vi "get integrated iq from h5.vi"(8 "error in (no error)":errorcluster, 11 "path":path=path "C:/Users/dvh-collab-user/Desktop/20230313 Robert sample/tmp.hdf5") -> (0 "error out":errorcluster, 3 "Data out":dbl[][](array[numeric]))   [LabVIEW 2023]
uses:
  <vilib>/UPVI/lvhdf5/library.llb/HDF5 Ref.ctl
  <vilib>/UPVI/lvhdf5/dataset.llb/Read Dataset and All Attributes.xnode
  <vilib>/Utility/miscctls.llb/LVRectTypeDef.ctl
  <vilib>/UPVI/lvhdf5/file.llb/H5Fopen.vi
  <vilib>/UPVI/lvhdf5/group.llb/H5G_obj_t.ctl
  <vilib>/UPVI/lvhdf5/dataset.llb/LVH5D Operation.ctl
  <vilib>/UPVI/lvhdf5/file.llb/LVH5F Operation.ctl
  <vilib>/UPVI/lvhdf5/utility.llb/Select HDF5 Dialog.vi
  <vilib>/UPVI/lvhdf5/utility.llb/Select HDF5 Dialog (File and Object).vi
  <vilib>/UPVI/lvhdf5/utility.llb/Select HDF5 Dialog (Object Only).vi
  <vilib>/UPVI/lvhdf5/identifier.llb/Not an HDF5 Refnum Constant.vi
  <vilib>/UPVI/lvhdf5/dataset.llb/Simple H5Dread (Variant).vi
  <vilib>/UPVI/lvhdf5/dataset.llb/OpenCreateReplace Dataset.vi
  <vilib>/UPVI/lvhdf5/dataset.llb/H5Dget_space.vi
  <vilib>/UPVI/lvhdf5/dataspace.llb/H5Sget_simple_extent_dims.vi
  <vilib>/UPVI/lvhdf5/dataspace.llb/H5Sselect_hyperslab.vi
  <vilib>/UPVI/lvhdf5/dataset.llb/H5Dread (Variant).vi
  <vilib>/UPVI/lvhdf5/attribute.llb/private/LVH5AreadWDTAttrs.vi
  <vilib>/UPVI/lvhdf5/dataspace.llb/H5Sclose.vi
  <vilib>/Utility/error.llb/Error Cluster From Error Code.vi
  <vilib>/UPVI/lvhdf5/attribute.llb/Attribute Array to Cluster.xnode
  <vilib>/UPVI/lvhdf5/attribute.llb/Read Multiple Attributes (Variant).vi
  <vilib>/UPVI/lvhdf5/dataset.llb/H5Dclose.vi
  <vilib>/Utility/Data Type/Get Type Information.vi
  <vilib>/Utility/Data Type/NI_Data Type.lvlib
  <vilib>/Utility/Data Type/Get Cluster Information.vi
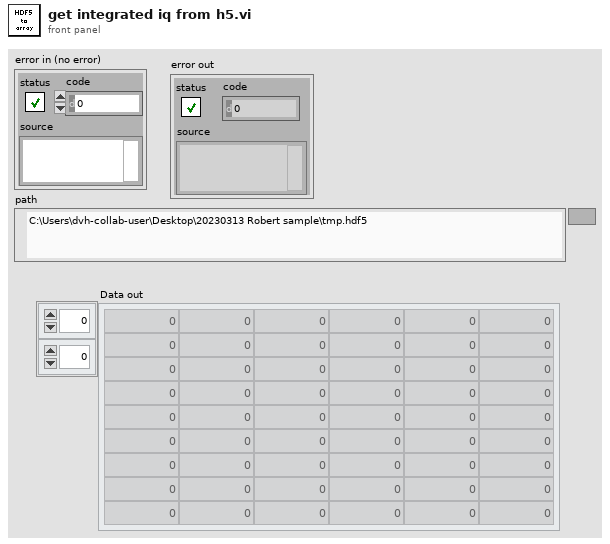
[diagram p1: front panel]
types:
  T1 = typedef "HDF5 Ref.ctl" = refnum<k1>
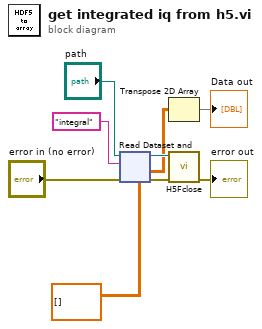
[diagram p0: block diagram]
diagram:
  n1 = xnode "Read Dataset and"("Dataset Path"="integral", "error in (no error)"="error in (no error)", "HDF5 Path or Ref"="path", "Data"=dbl[][] []) -> ("HDF5 Ref out"=w6:T1, "error out"=w5:errorcluster, "Data out"=w2:dbl[][])  [unwired: 2 in, 3 out]
  n2 = Transpose 2D Array(2D array=w2) -> (transposed array=→"Data out":dbl[][])
  n3 = call <vilib>:"H5Fclose.vi"("error in (no error)"=w5, "HDF5 Ref"=w6) -> ("error out"=→"error out":errorcluster)  [unwired: 7 in]
